vi "Read Configuration.vi"(8 "error in (no error)":errorcluster, 9 "Default Values":variant[](array[variant]), 10 "URIs":string[](array[string]), 11 "Attribute.Config in":refnum<class "Attribute.Config.lvclass">) -> (0 "error out":errorcluster, 1 "Values":variant[](array[variant]), 2 "URIs dup":string[](array[string]), 3 "Attribute.Config out":refnum<class "Attribute.Config.lvclass">)   [LabVIEW 2013, in "Attribute.Config.lvclass"]
uses:
  Attribute.Config.lvclass
  Attribute.Config.lvclass/Attribute.Config.ctl
  <vilib>/LabVIEW Open Source/Configuration Manager/Manager/ConfigManager.lvclass
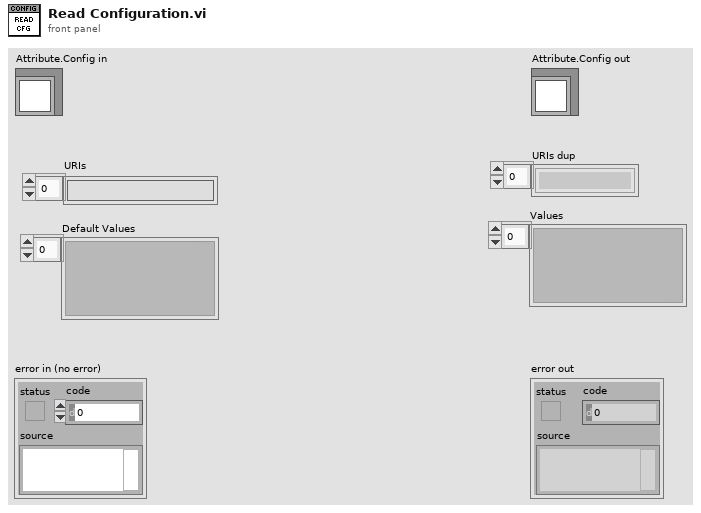
[diagram p1: front panel]
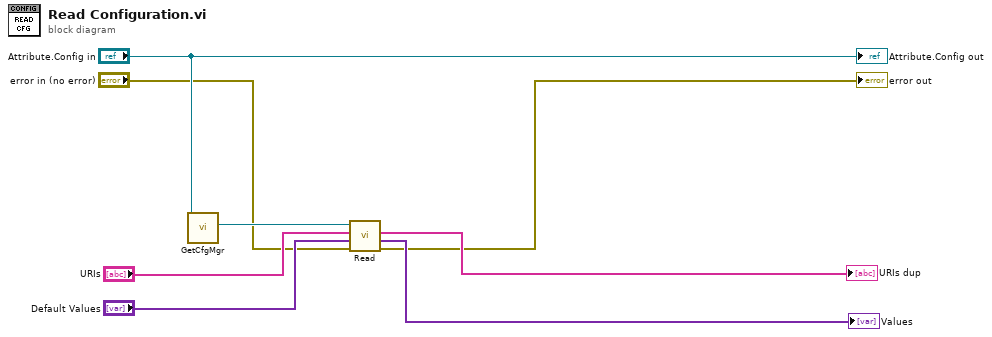
[diagram p0: block diagram]
diagram:
  n1 = call "GetCfgMgr.vi"("Attribute.Config in"="Attribute.Config in") -> ("CfgMgr"=w7:refnum<class "ConfigManager.lvclass">)  [unwired: 9 in, 1 out]
  n2 = call <vilib>:"Read.vi"("error in (no error)"="error in (no error)", "Default Values"="Default Values", "keys in"="URIs", "ConfigManager in"=w7) -> ("error out"=→"error out":errorcluster, "Values"=→"Values":variant[], "keys"=→"URIs dup":string[])  [unwired: 4 in, 1 out]
  "Attribute.Config out" <- "Attribute.Config in"
